vi "PXI_Host_Cluster_Read_OldMethod_Benchmark.vi"() -> ()   [LabVIEW 2018]
uses:
  <vilib>/Platform/TimedLoop/XDataNode/timing_clust.ctl
  <vilib>/Platform/TimedLoop/XDataNode/nitl_modes.ctl
  <vilib>/Platform/TimedLoop/XDataNode/wakeup.ctl
  <vilib>/addons/FPGA Advanced Session Resources/LVFPGA Adv Session Resources/OpenByNameSubVI.vi
  <vilib>/rvi/interface/common/dynamic/niFpgaEscapeDelimiterAndNull.vi
  <vilib>/Utility/error.llb/Error Cluster From Error Code.vi
  <vilib>/rvi/errors/niLvFpgaAdjustHostInterfaceError.vi
  <vilib>/FPGAPlugInAG/Dynamic/niLvFpga_Close_Dynamic.vi
  <vilib>/addons/FPGA Advanced Session Resources/LVFPGA Adv Session Resources/OpenByName.xnode
  <vilib>/platform/TimedLoop/XDataNode/XDataNode.xnode
  <vilib>/rvi/interface/nirviReadWriteControl/nirviReadWriteControl.xnode
  <vilib>/rvi/interface/nirviCloseFPGA/nirviCloseFPGA.xnode
  NiFpgaLv.dll
  <vilib>/rvi/interface/Simulation/niFpgaSimulationCallBeginRW.vi
  <vilib>/addons/FPGA Advanced Session Resources/LVFPGA Adv Session Resources/LVFPGAAdvSessionResources.lvlib
  <vilib>/Platform/TimedLoop/XDataNode/XDNodeRunTimeDep.lvlib
panel:
  out "Waveform Graph":dbl[](graph)
  out "Standard Dev":dbl
  out "Execution time (s)":dbl
  out "Maximum(s)":dbl
  out "error out":errorcluster
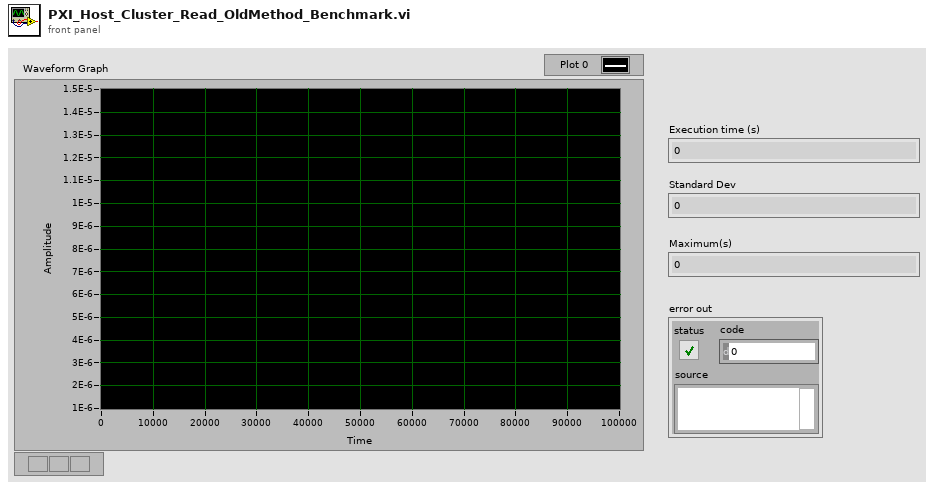
[diagram p1: front panel]
types:
  T1 = typedef "XDNodeRunTimeDep.lvlib/timing_clust.ctl" = cluster{"Expected End [f-1]":u64, "Actual End [f-1]":u64, "Finished Late? [f-1]":bool, "Expected End [i-1]":u64, "Actual End [i-1]":u64, "Finished Late? [i-1]":bool, "Expected Start [i]":u64, "Actual Start [i]":u64, "Expected Start [f]":u64, "Actual Start [f]":u64, "Source Name":string, "Structure Name":string, "Period":i64, "Deadline":i64, "Offset":i64, "Start":i64, "Priority":i32, "Timeout":i32, "Mode":T2, "Wakeup Reason":T3, "Error":errorcluster, "Source Type":string, "Secondary Source Type":string, "Global End Time":u64, "Global Start Time":u64, "Frame Duration":u64, "Iteration Duration":u64, "Assigned CPU":i32, "I/O Scan Engine Mode":u32}
  T2 = typedef "XDNodeRunTimeDep.lvlib/nitl_modes.ctl" = enum32{"No Change", "Process missed periods, maintain original phase", "Discard missed periods, maintain original phase", "Process missed periods, ignore original phase", "Discard missed periods, ignore original phase"}
  T3 = typedef "XDNodeRunTimeDep.lvlib/wakeup.ctl" = enum32{"Normal", "Aborted", "Asynchronous wakeup", "Timing source error", "Timed loop error", "Timeout"}
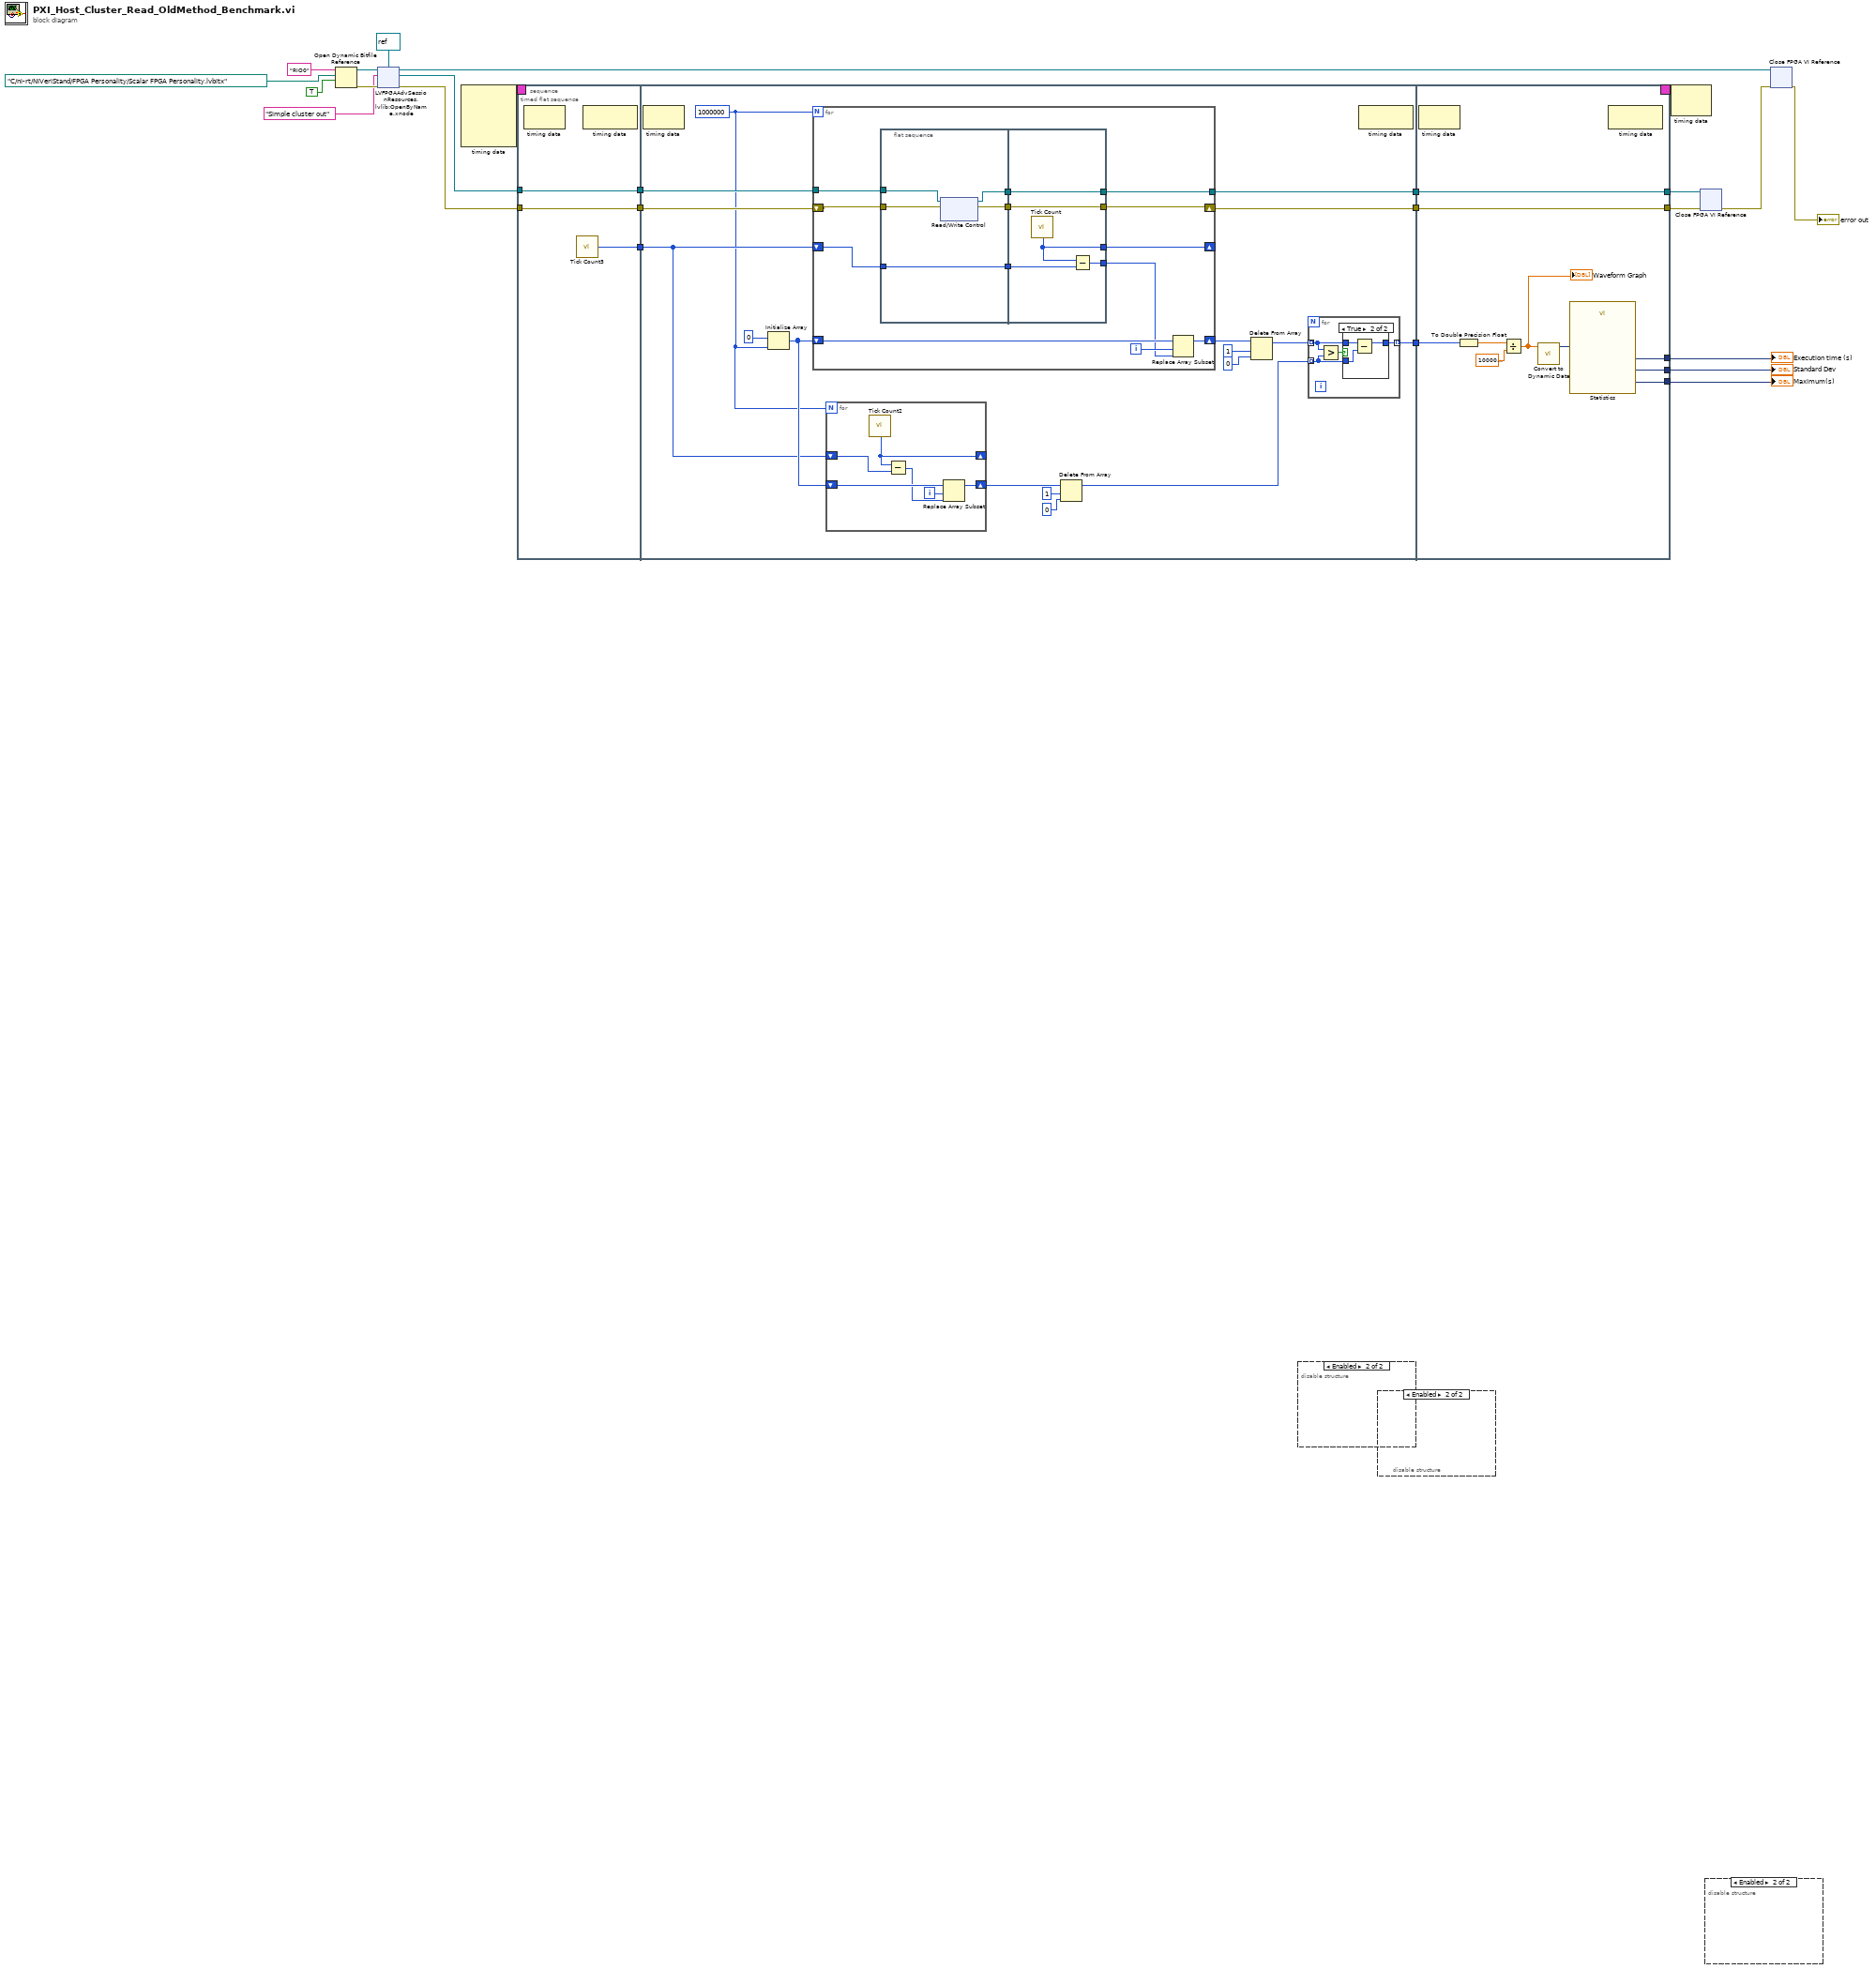
[diagram p0: block diagram]
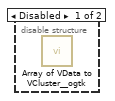
[diagram p3: hidden frame]
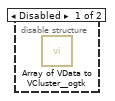
[diagram p4: hidden frame]
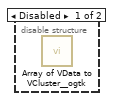
[diagram p5: hidden frame]
diagram:
  n1 = Open Dynamic Bitfile Reference(0:"RIO0" ("device address"), 1:path "C:/ni-rt/NIVeriStand/FPGA Personality/Scalar FPGA Personality.lvbitx" ("bitfile path"), 2:TRUE ("run when loaded (T)")) -> (5:w8:refnum<k20>, 8:w10:errorcluster)  [unwired: 2 in]
  n2 = xnode "LVFPGAAdvSessionResources.lvlib:OpenByName.xnode"("FPGA VI Reference in"=w8, "Resource name in"="Simple cluster out", "Single resource reference type in"=refnum<k20> refnum ("Type"), "Error in"=w10) -> ("Single resource reference out"=w5:refnum<k20>, "Error out"=w4:errorcluster, "FPGA VI Reference out"=w6:refnum<k20>)
  n3 = node-c288() -> (w19:T1)  [unwired: 4 in]
  n4 = timed-sequence {
    timing: w19 -> [_]
    timing-out: [_] -> w18
    tunnel: w5 -> [w32]
    tunnel: w4 -> [w31]
    tunnel: [w30] -> w3
    tunnel: [w24] -> w16
    tunnel: [w23] -> w15
    tunnel: [w22] -> w14
    tunnel: [w21] -> w1
    n5 = timed-flat-sequence {
      tunnel: w31 -> [w34]
      tunnel: w32 -> [w35]
      tunnel: [w35] -> w29
      tunnel: [w34] -> w28
      tunnel: [w33] -> w27
      tunnel: w29 -> [w54]
      tunnel: w28 -> [w53]
      tunnel: w27 -> [w40]
      tunnel: [w52] -> w26
      tunnel: [w41] -> w25
      tunnel: [w38] -> w20
      tunnel: [w103] -> w30
      tunnel: w26 -> [w103]
      tunnel: w25 -> [w99]
      tunnel: [w98] -> w24
      tunnel: [w97] -> w23
      tunnel: [w96] -> w22
      tunnel: [w94] -> w21
      tunnel: w20 -> [w94]
      frame #0 {
        n6 = node-c288() -> ()  [unwired: 1 in, 1 out]
        n7 = call "Tick Count3"() -> ("Tick Count(Ticks)"=w33:u32)
        n8 = node-c288() -> ()  [unwired: 1 in, 1 out]
      }
      frame #1 {
        w39 = 1000000
        n9 = node-c288() -> ()  [unwired: 1 in, 1 out]
        n10 = Initialize Array(u32 0 ("Tick Count(uSec)"), w39) -> (w50:u32[])
        n11 = for {
          N: w39 -> [_]
          tunnel: w54 -> [w76]
          shift-right: [w67] -> w52
          shift-left: w53 -> [w75]
          shift-right: [w72] -> w44
          shift-left: w50 -> [w74]
          shift-right: [w69] -> _
          shift-left: w40 -> [w71]
          tunnel: [w65] -> w38
          i -> [w73]
          n12 = flat-sequence {
            tunnel: [w82] -> w77
            tunnel: w71 -> [w82]
            tunnel: w76 -> [w80]
            tunnel: w75 -> [w79]
            tunnel: [w81] -> w68
            tunnel: [w78] -> w66
            tunnel: w77 -> [w87]
            tunnel: [w86] -> w70
            tunnel: [w85] -> w69
            tunnel: w68 -> [w84]
            tunnel: [w84] -> w67
            tunnel: w66 -> [w83]
            tunnel: [w83] -> w65
            frame #0 {
              n13 = xnode "Read/Write Control"("FPGA VI Reference In"=w80, "error in"=w79) -> ("FPGA VI Reference Out"=w78:refnum<k20>, "error out"=w81:errorcluster)  [unwired: 1 out]
            }
            frame #1 {
              n14 = call "Tick Count"() -> ("Tick Count(Ticks)"=w85:u32)
              n15 = Subtract(x=w85, y=w87) -> (x-y=w86:u32)
            }
          }
          n16 = Replace Array Subset(array=w74, new element=w70, index=w73) -> (w72:u32[])
        }
        n17 = for {
          N: w39 -> [_]
          shift-right: [w88] -> w47
          shift-left: w50 -> [w91]
          shift-right: [w93] -> _
          shift-left: w40 -> [w92]
          i -> [w89]
          n18 = call "Tick Count2"() -> ("Tick Count(Ticks)"=w93:u32)
          n19 = Subtract(x=w93, y=w92) -> (x-y=w90:u32)
          n20 = Replace Array Subset(array=w91, new element=w90, index=w89) -> (w88:u32[])
        }
        n21 = Delete From Array(array=w47, length=1, index=0) -> (array with subset deleted=w42:u32[])  [unwired: 1 out]
        n22 = Delete From Array(array=w44, length=1, index=0) -> (array with subset deleted=w43:u32[])  [unwired: 1 out]
        n23 = for {
          tunnel: [w60] -> w41 mode=indexing
          tunnel: w43 -> [w59] mode=indexing
          tunnel: w42 -> [w58] mode=indexing
          n24 = Greater?(x=w59, y=w58) -> (0:w57:bool)
          n25 = case shown="True" w57 {
            tunnel: w59 -> [w61 w64]
            tunnel: w58 -> [_ w63]
            tunnel: [w61 w62] -> w60
            frame False {
            }
            frame True {
              n26 = Subtract(x=w64, y=w63) -> (x-y=w62:u32)
            }
          }
        }
        n27 = node-c288() -> ()  [unwired: 1 in, 1 out]
      }
      frame #2 {
        n28 = node-c288() -> ()  [unwired: 1 in, 1 out]
        n29 = To Double Precision Float(number=w99) -> (double precision float=w102:dbl[])
        n30 = Divide(x=w102, y=1000000000.0) -> (x/y=w95:dbl[])
        "Waveform Graph" <- w95
        n31 = call "Convert to Dynamic Data"("Array"=w95) -> ("Dynamic Data Type"=w100:dynamicdata)  [unwired: 3 in]
        n32 = call "Statistics"("Signals"=w100) -> ("Standard Dev"=w97:dynamicdata, "Arithmetic Mean"=w98:dynamicdata, "Maximum"=w96:dynamicdata)  [unwired: 23 in, 1 out]
        n33 = node-c288() -> ()  [unwired: 1 in, 1 out]
      }
    }
  }
  "Maximum(s)" <- w14
  "Execution time (s)" <- w16
  "Standard Dev" <- w15
  n34 = disable-structure shown="Enabled" {
    frame Disabled {
      n35 = call <userlib>:"Array of VData to VCluster__ogtk.vi"() -> ()  [unwired: 10 in, 2 out]
    }
    frame Enabled {
    }
  }
  n36 = disable-structure shown="Enabled" {
    frame Disabled {
      n37 = call <userlib>:"Array of VData to VCluster__ogtk.vi"() -> ()  [unwired: 10 in, 2 out]
    }
    frame Enabled {
    }
  }
  n38 = node-c288(w18) -> ()  [unwired: 1 out]
  n39 = xnode "Close FPGA VI Reference"("FPGA VI Reference In"=w1, "error in"=w3) -> ("error out"=w2:errorcluster)
  n40 = disable-structure shown="Enabled" {
    frame Disabled {
      n41 = call <userlib>:"Array of VData to VCluster__ogtk.vi"() -> ()  [unwired: 10 in, 2 out]
    }
    frame Enabled {
    }
  }
  n42 = xnode "Close FPGA VI Reference"("FPGA VI Reference In"=w6, "error in"=w2) -> ("error out"=→"error out":errorcluster)
